vi "GetFeaturePropertyName.vi"(9 "unit":string, 10 "metric name":string) -> (1 "tdms unit value":string, 2 "display name":string, 3 "tdms property name":string)   [LabVIEW 2017, in "Tdms.lvlib"]
uses:
  <vilib>/addons/InsightCM/Utilities/Tdms/Tdms.lvlib
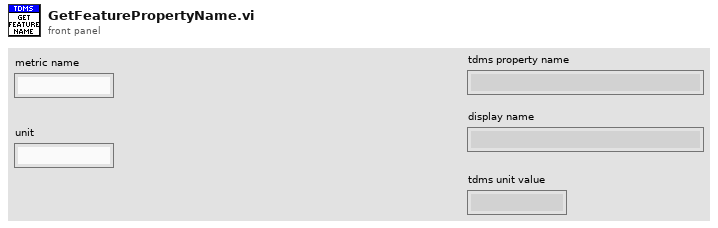
[diagram p1: front panel]
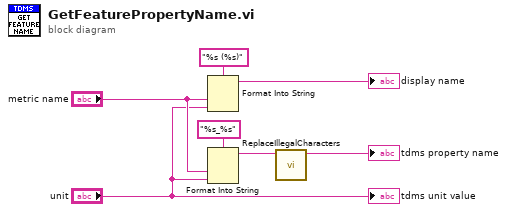
[diagram p0: block diagram]
diagram:
  n1 = Format Into String(format string="%s (%s)", "metric name", "unit") -> (resulting string=→"display name":string)  [unwired: 2 in, 1 out]
  n2 = Format Into String(format string="%s_%s", "metric name", "unit") -> (resulting string=w4:string)  [unwired: 2 in, 1 out]
  n3 = call <vilib>:"ReplaceIllegalCharacters.vi"("input string"=w4) -> ("result string"=→"tdms property name":string)  [unwired: 10 in]
  "tdms unit value" <- "unit"
